vi "Write-Read Byte Array Demo - TESTS.vi"() -> ()   [LabVIEW 2017]
panel:
  out "FT_Status":u64
  out "Device Description":string
  in  "Device Index":u32
  # "Enter values in Write Buffer and run program.  \nWith a loop-back connector, the data is read back into the Read Buffer."
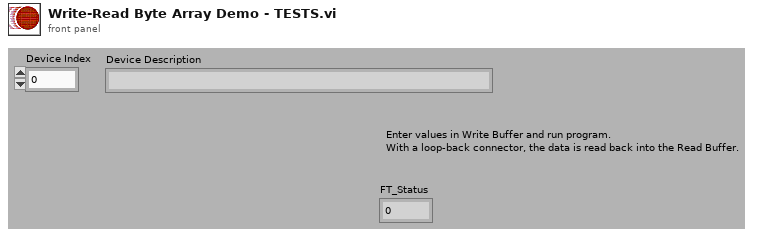
[diagram p1: front panel]
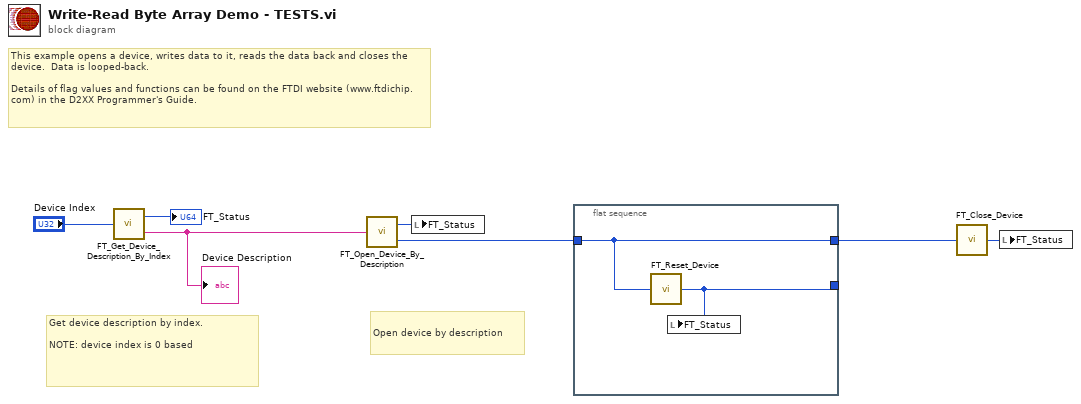
[diagram p0: block diagram]
diagram:
  # "Open device by description"
  # "Get device description by index.\n\nNOTE: device index is 0 based"
  # "This example opens a device, writes data to it, reads the data back and closes the device.  Data is looped-back.\n\nDetails of flag values and functions can be found on the FTDI website (www.ftdichip.com) in the D2XX Programmer's Guide."
  n1 = call "FT_Get_Device_Description_By_Index.vi"("Device Index"="Device Index") -> ("FT_Status"=→"FT_Status":u64, "Device Description"=w7:string)
  "Device Description" <- w7
  n2 = call "FT_Open_Device_By_Description.vi"("Device Description"=w7) -> ("FT_Status"=w4:u64, "Handle"=w2:u64)
  n3 = local write "FT_Status"(w4) -> ()
  n4 = flat-sequence {
    tunnel: w2 -> [w8]
    tunnel: [w9] -> _
    tunnel: [w8] -> w1
    frame #0 {
      n5 = call "FT_Reset_Device.vi"("Handle"=w8) -> ("FT_Status"=w9:u32)
      n6 = local write "FT_Status"(w9) -> ()
    }
  }
  n7 = call "FT_Close_Device.vi"("Handle"=w1) -> ("FT_Status"=w3:u64)
  n8 = local write "FT_Status"(w3) -> ()
